vi "Command2ControlValues.vi"(8 "error in":errorcluster, 11 "Command":string) -> (0 "error out":errorcluster, 1 "(S)Selected/(N)Unselected":bool, 2 "(N)ON/(F)OFF":bool, 3 "Intensity":u8(slide) step=1 scale=0.0..100.0)   [LabVIEW 2025]
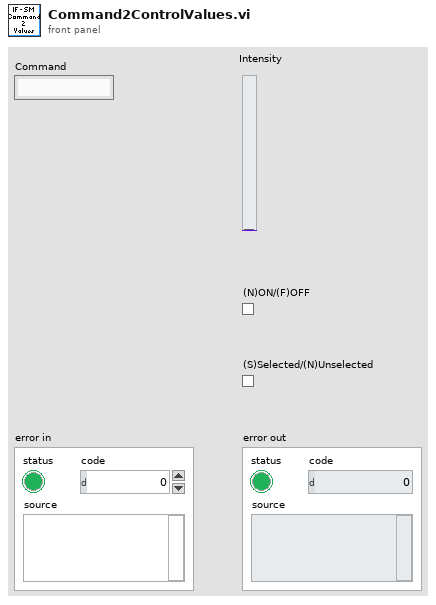
[diagram p1: front panel]
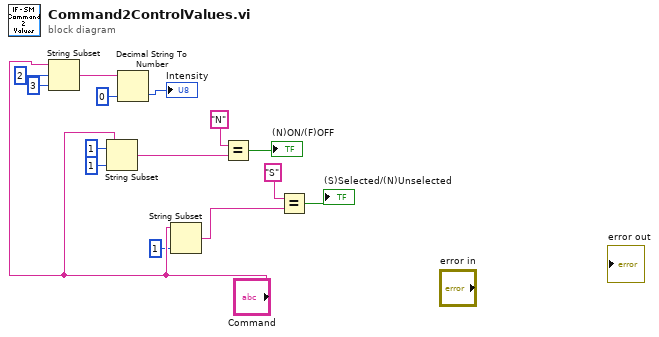
[diagram p0: block diagram]
diagram:
  n1 = String Subset(string="Command", offset (0)=2, length (rest)=3 ("length (rest)")) -> (substring=w7:string)
  n2 = String Subset(string="Command", offset (0)=1, length (rest)=1 ("length (rest)")) -> (substring=w11:string)
  n3 = Decimal String To Number(string=w7, default (0L)=u8 0 ("default (0 I32)")) -> (number=→"Intensity":u8)  [unwired: 1 in, 1 out]
  n4 = String Subset(string="Command", length (rest)=1 ("length (rest)")) -> (substring=w13:string)  [unwired: 1 in]
  n5 = Equal?(x="N", y=w11) -> (x = y?=→"(N)ON/(F)OFF":bool)
  n6 = Equal?(x="S", y=w13) -> (x = y?=→"(S)Selected/(N)Unselected":bool)
